vi "run_program.vi"(0 "program id in":u32, 1 "operation":T1(ring), 3 "data in":string) -> (5 "program id out":u32, 6 "bytes read":i32, 7 "data out":string)   [LabVIEW 2015]
doc: "Copyright (c) 2018 Frans Korhonen, Institute for Atmospheric and Earth System Research / Physics, Faculty of Science, University of Helsinki, Finland\n\nThis file is part of MeasGUI.\n\nThis Source Code Form is subject to the terms of the Mozilla Public\nLicense, v. 2.0. If a copy of the MPL was not distributed with this\n file, You can obtain one at http://mozilla.org/MPL/2.0/."
panel:
  out "VI or executable installation directory":path
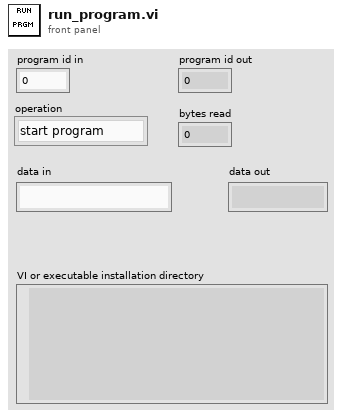
[diagram p1: front panel]
types:
  T1 = enum16{"start program", "write", "read", "terminate", "clear buffer"}
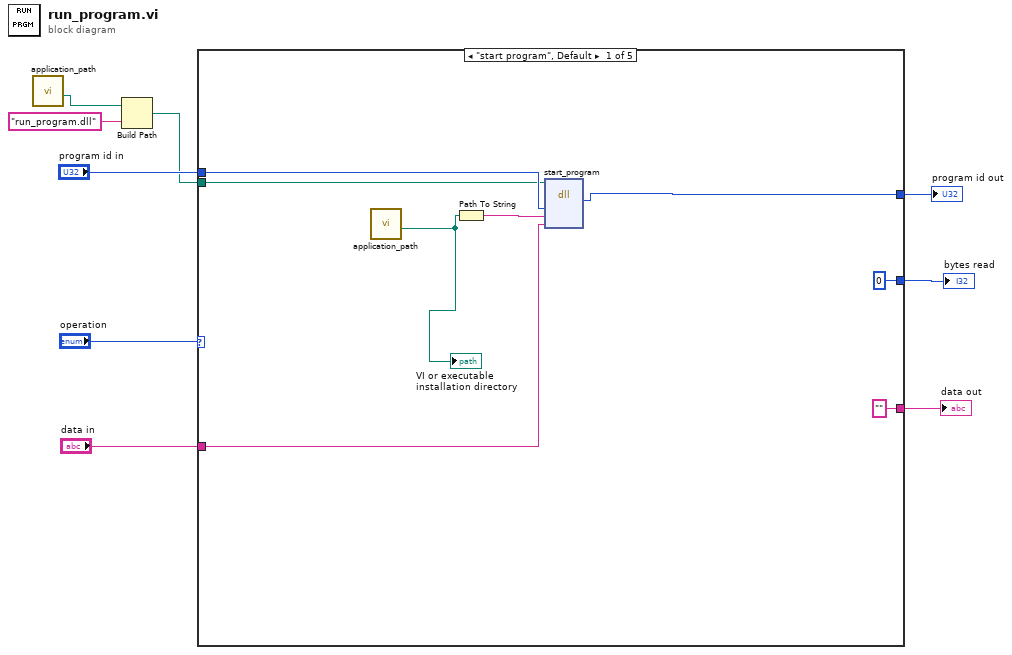
[diagram p0: block diagram]
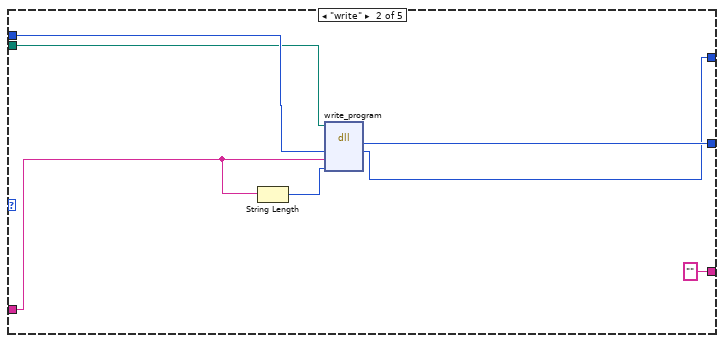
[diagram p2: hidden frame]
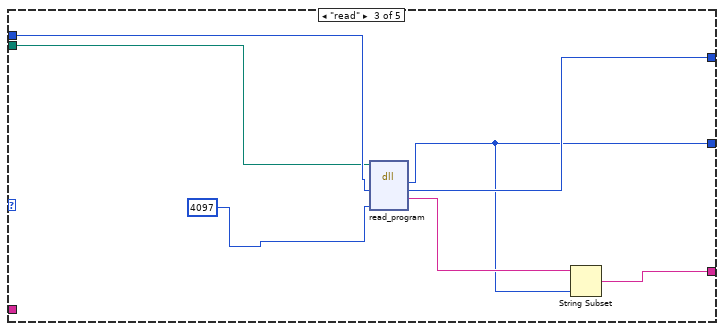
[diagram p3: hidden frame]
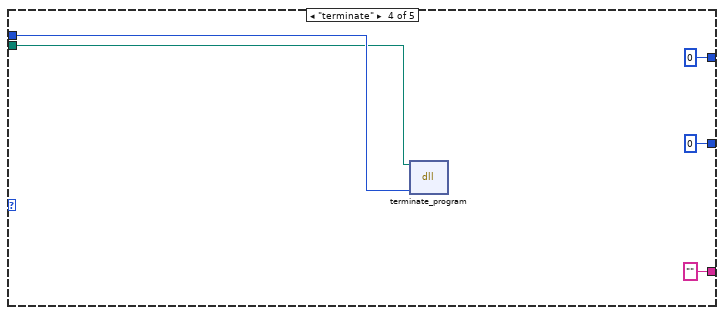
[diagram p4: hidden frame]
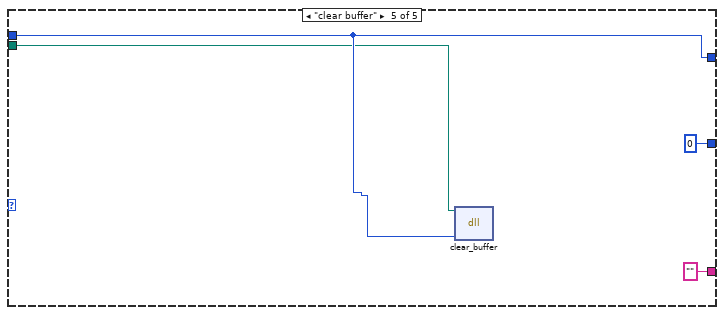
[diagram p5: hidden frame]
diagram:
  n1 = call "application_path.vi"() -> ("path"=w3:path)  [unwired: 11 in]
  n2 = Build Path(base path=w3, name or relative path="run_program.dll") -> (appended path=w2:path)
  n3 = case shown="\"start program\", Default" "operation" {
    tunnel: [w13 w22 w30 u32 0 ("program") w38] -> w5
    tunnel: "data in" -> [w16 w21 _ _ _]
    tunnel: [0 w23 w27 0 0 ("return type")] -> w7
    tunnel: "program id in" -> [w12 w20 w31 w36 w38]
    tunnel: ["" ("buffer") "" ("buffer") w26 "" ("buffer") "" ("buffer")] -> w6
    tunnel: w2 -> [w11 w18 w29 w32 w37]
    frame "start program", Default {
      n4 = call "application_path.vi"() -> ("path"=w10:path)  [unwired: 11 in]
      "VI or executable installation directory" <- w10
      n5 = Path To String(path=w10) -> (string=w17:string)
      n6 = dll-call lib="C:/hyapp/tools/channel_system_windows/run_program.dll" fn="start_program"(path in=w11, "program"=w12, "work_dir"=w17, "program_command"=w16) -> ("return type"=w13:u32)  [unwired: 5 in, 2 out]
    }
    frame "write" {
      n7 = String Length(string=w21) -> (length=w24:i32)
      n8 = dll-call lib="run_program.dll" fn="write_program"(path in=w18, "program"=w20, "buffer"=w21, "buffer_len"=w24) -> ("return type"=w23:i32, "program"=w22:u32)  [unwired: 4 in, 2 out]
    }
    frame "read" {
      n9 = dll-call lib="run_program.dll" fn="read_program"(path in=w29, "program"=w31, "buffer_len"=u32 4097 ("dimension size")) -> ("return type"=w27:i32, "program"=w30:u32, "buffer"=w28:string)  [unwired: 4 in, 2 out]
      n10 = String Subset(string=w28, length (rest)=w27) -> (substring=w26:string)  [unwired: 1 in]
    }
    frame "terminate" {
      n11 = dll-call lib="run_program.dll" fn="terminate_program"(path in=w32, "program"=w36) -> ()  [unwired: 4 in, 2 out]
    }
    frame "clear buffer" {
      n12 = dll-call lib="run_program.dll" fn="clear_buffer"(path in=w37, "program"=w38) -> ()  [unwired: 4 in, 2 out]
    }
  }
  "program id out" <- w5
  "data out" <- w6
  "bytes read" <- w7
